vi "SetParam.vi"(8 "error in (no error)":errorcluster caption="entrée d'erreur (pas d'erreur)", 10 "hinge_loss":cluster{"labels":i32[], "sample_weight":dbl[]}, 11 "Hinge_Loss.lvclass":refnum<class "Hinge_Loss.lvclass">) -> (0 "error out":errorcluster caption="sortie d'erreur", 3 "Hinge_Loss.lvclass":refnum<class "Hinge_Loss.lvclass">)   [LabVIEW 2020, in "Hinge_Loss.lvclass"]
doc: "Set Parameters"
uses:
  Hinge_Loss.lvclass
  Hinge_Loss.lvclass/Hinge_Loss.ctl
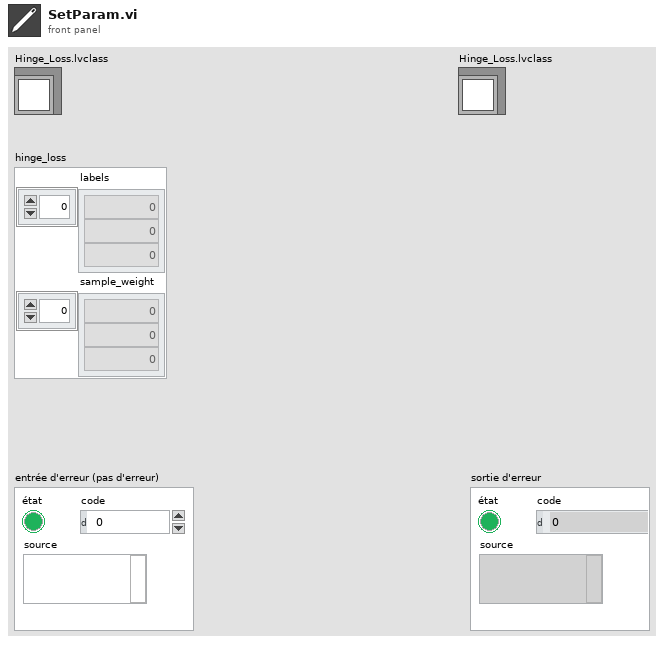
[diagram p1: front panel]
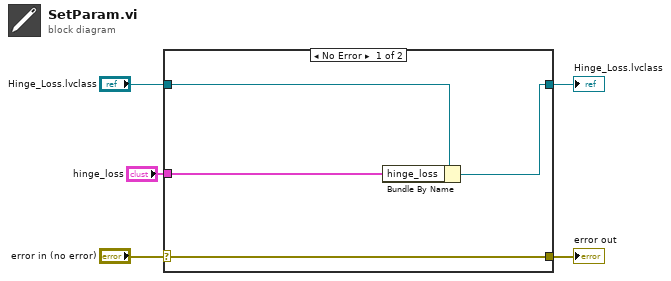
[diagram p0: block diagram]
diagram:
  n1 = case shown="No Error" "error in (no error)" {
    selector: "error in (no error)" -> [w9 w10]
    tunnel: [w9 w10] -> w4
    tunnel: [w7 w11] -> w2
    tunnel: "Hinge_Loss.lvclass" -> [w8 w11]
    tunnel: "hinge_loss" -> [w6 _]
    frame No Error {
      n2 = Bundle By Name(cluster=w8, "hinge_loss"=w6) -> (w7:refnum<class "Hinge_Loss.lvclass">)
    }
    frame Error {
    }
  }
  "error out" <- w4
  "Hinge_Loss.lvclass" <- w2
